vi "getConnectFlags.vi"(11 "CONNECT in":refnum<class "CONNECT.lvclass">) -> (2 "Connect Flags":T1, 3 "CONNECT out":refnum<class "CONNECT.lvclass">)   [LabVIEW 2013, in "CONNECT.lvclass"]
uses:
  CONNECT.lvclass
  ConnectFlags -- cluster.ctl
  ControlPacket/ControlPacket.lvclass/ControlPacket.ctl
  ControlPacket/ControlPacket.lvclass
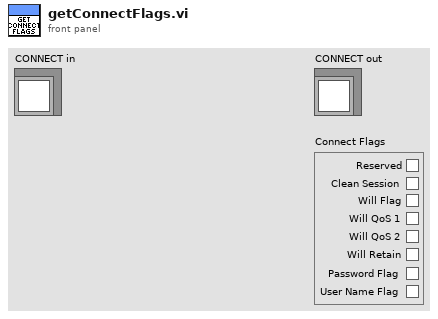
[diagram p1: front panel]
types:
  T1 = typedef "CONNECT.lvclass/ConnectFlags -- cluster.ctl" = cluster{"Reserved":bool, "Clean Session":bool, "Will Flag":bool, "Will QoS 1":bool, "Will QoS 2":bool, "Will Retain":bool, "Password Flag":bool, "User Name Flag":bool}
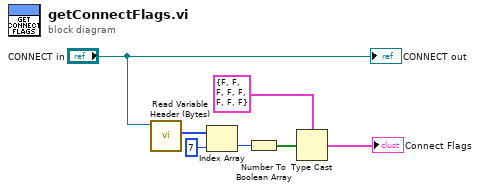
[diagram p0: block diagram]
diagram:
  n1 = call "Read Variable Header (Bytes).vi"("ControlPacket in"="CONNECT in") -> ("Variable Header (Bytes)"=w6:u8[])  [unwired: 9 in, 1 out]
  n2 = Index Array(array=w6, index=7) -> (element=w4:u8)
  n3 = Number To Boolean Array(number=w4) -> (Boolean array=w3:bool[])
  n4 = Type Cast(type=T1 {"Reserved"=FALSE, "Clean Session"=FALSE, "Will Flag"=FALSE, "Will QoS 1"=FALSE, "Will QoS 2"=FALSE, "Will Retain"=FALSE, "Password Flag"=FALSE, "User Name Flag"=FALSE} ("Connect Flags"), x=w3) -> (*(type *) &x=→"Connect Flags":T1)
  "CONNECT out" <- "CONNECT in"
